vi "GFITS_GetEarlyHeaders.vi"(0 "file":path, 1 "Database RefNum in":T1, 11 "error in (no error)":errorcluster, 12 "def_timing":string="after") -> (15 "error out":errorcluster)   [LabVIEW 2016]
uses:
  DBSHAND/private/vis/DatabaseHand_RefNum.ctl
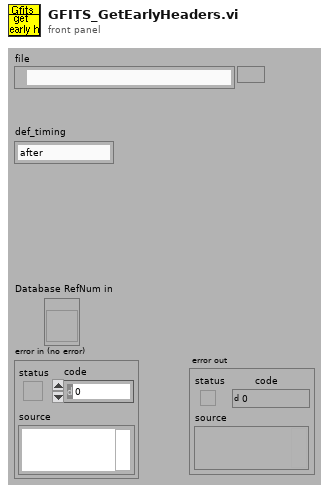
[diagram p1: front panel]
types:
  T1 = typedef "DatabaseHand_RefNum.ctl" = refnum<vi>
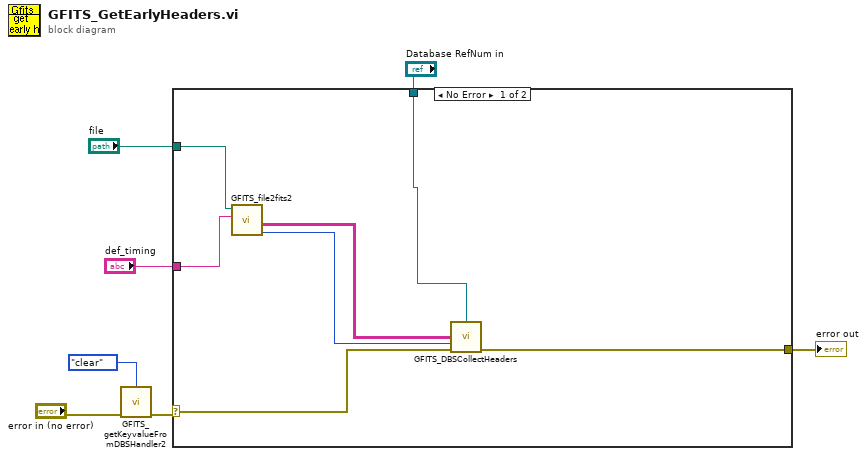
[diagram p0: block diagram]
diagram:
  n1 = call "GFITS_getKeyvalueFromDBSHandler2.vi"("action"=enum16{"get", "clear"}."clear", "error in (no error)"="error in (no error)") -> ("error out"=w2:errorcluster)  [unwired: 7 in, 6 out]
  n2 = case shown="No Error" w2 {
    selector: w2 -> [w10 w15]
    tunnel: "file" -> [w14 _]
    tunnel: "def_timing" -> [w13 _]
    tunnel: [w12 w15] -> w4
    tunnel: "Database RefNum in" -> [w11 _]
    frame No Error {
      n3 = call "GFITS_file2fits2.vi"("def_timing"=w13, "file"=w14) -> ("number of before keywords"=w9:i32, "before Keywords"=w8:string[][])  [unwired: 8 out]
      n4 = call "GFITS_DBSCollectHeaders.vi"("Database RefNum in"=w11, "Keywords"=w8, "numer of keywords"=w9, "error in (no error)"=w10) -> ("error out"=w12:errorcluster)  [unwired: 11 out]
    }
    frame Error {
    }
  }
  "error out" <- w4
